vi "TTA_MATLAB_RFICSetDGAttTest.vi"(0 "Complete Settings Cluster":T2, 1 "Instrument Cluster In":T1, 5 "Sub-Function Name":string, 7 "Test Group":string, 11 "error in":errorcluster) -> (6 "SubTestSuccess":dbl[](array[numeric]), 12 "Instrument Cluster Out":T1, 15 "error out":errorcluster)   [LabVIEW 2016]
uses:
  TTA_Controls/TTA_Control_Complete_Settings_Cluster.ctl
  TTA_Controls/TTA_Control_Instrument_Cluster.ctl
  TTA_Globals/TTA_Global_Complete_Settings.vi
panel:
  out "Tx Result":cluster{"TX1":dbl[], "TXx3":dbl[]}[](array[cluster])
  out "Test Status":string
  out "DigAtt Min":dbl
  out "DigAtt Max":dbl
  out "Total RF Tx Loss (dB)":dbl
  out "Tx_Output_Power_Signal_Freq":dbl
  out "TxIF_Freq":dbl
  out "TxIF_Amp":dbl
  out "Tx IF\nOffset Array":dbl[](array[numeric])
  out "Sig Gen \nPower (dBm)":dbl
  out "Freq2":dbl
  out "BDSFreq":dbl
  out "Ref Level (dBm)":dbl
  out "RBW (Hz)":dbl
  out "Span (kHz)":dbl
  out "RFICs":i32[](array[numeric])
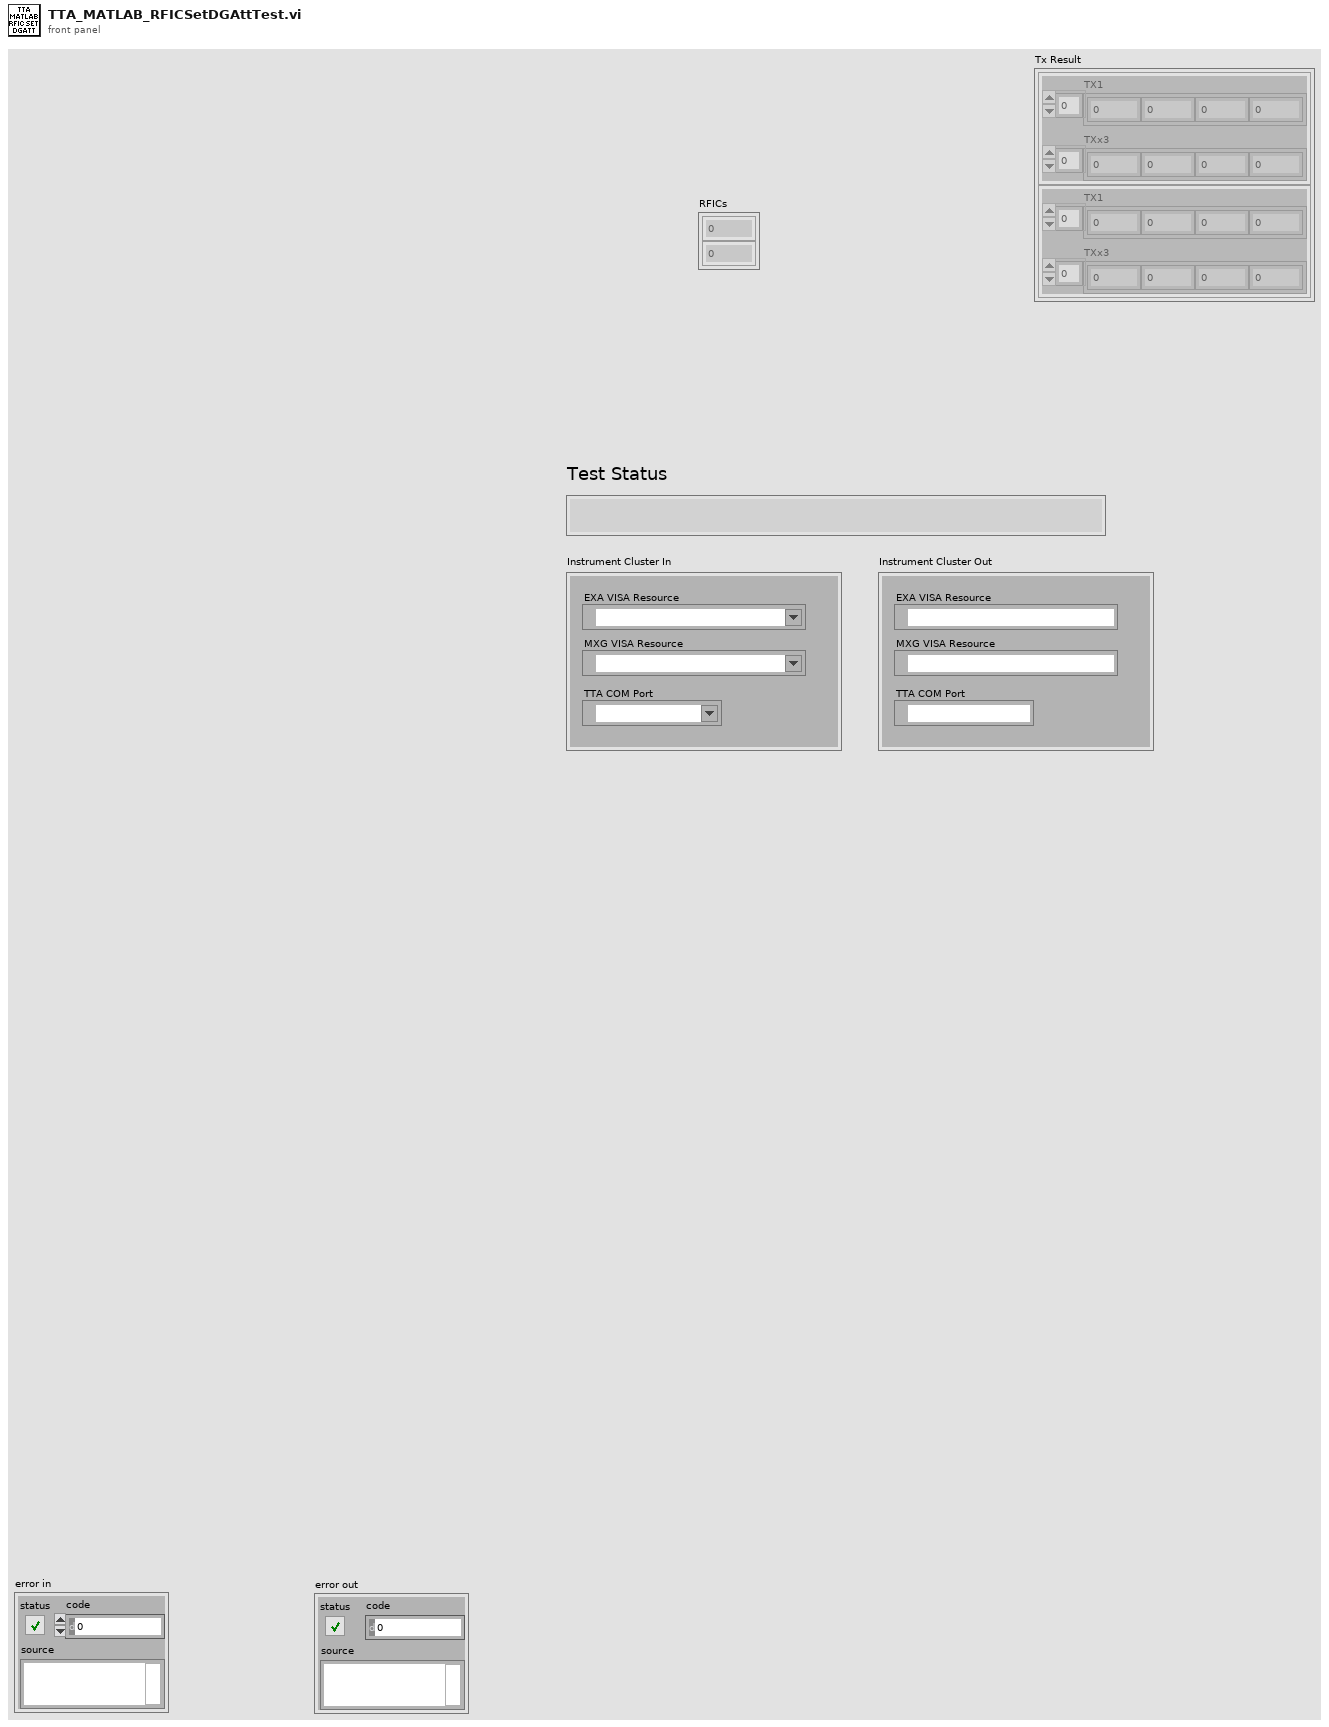
[diagram p1: front panel]
types:
  T1 = typedef "TTA_Control_Instrument_Cluster.ctl" = cluster{"EXA VISA Resource":refnum<visa-resource-name>, "MXG VISA Resource":refnum<visa-resource-name>, "TTA COM Port":refnum<visa-resource-name>}
  T2 = typedef "TTA_Control_Complete_Settings_Cluster.ctl" = cluster{"Brief Cluster":cluster{"STM Firmware File":string, "STM Firmware Address":string, "Required SW Version":string, "Template Used":string}, "Instrument Setting Cluster":cluster{"BDSFreq":dbl, "BDS Amp":dbl, "TxRFCal_Freq":dbl, "TxRFCal_Amp":dbl, "RxRFCal_Freq":dbl, "RxRFCal_Freq":dbl, "TxIF_Freq":dbl, "TxIF_Amp":dbl, "Tx_Output_Power_Signal_Freq":dbl, "Tx_ACPR_Signal_Freq":dbl, "Rx_RF_Freq":dbl, "Rx_RF_Amp":dbl, "Rx_Output_Power_Signal_Freq":dbl, "Rx_Output_Power_Sense_Freq":dbl}, "PAL Calibration\nInputs Cluster":cluster{"Amplitude Range\nMax(dBm)":dbl, "Amplitude Range\nMin(dBm)":dbl, "Amplitude Least\nCriteria (dBm)":dbl, "Frequency 1":dbl, "Frequency 2":dbl, "Frequency 3":dbl, "CAL Amplitude\nDecrement (dB)":dbl, "CAL Amplitude\nIncrement(dB)":dbl, "DownloadFile":string}, "TxOffset Cal Cluster":cluster{"Tx1 Offset (dB)":dbl, "Tx2 Offset (dB)":dbl, "Tx3 Offset (dB)":dbl, "Tx4 Offset (dB)":dbl, "Total RF Tx Loss (dB)":dbl}, "RxOffset Cal Cluster":cluster{"Rx1 Offset (dB)":dbl, "Rx2 Offset (dB)":dbl, "Rx3 Offset (dB)":dbl, "Rx4 Offset (dB)":dbl, "Total RF Rx Loss (dB)":dbl}, "TX Output Power Settings Cluster":cluster{"Frequency Sweep (MHz)":dbl[], "Sig Gen \nPower (dBm)":dbl, "Span (kHz)":dbl, "RBW (Hz)":dbl, "Ref Level (dBm)":dbl, "Low Power \nLimit":dbl, "High Power \nLimit":dbl, "DigAtt Max":dbl, "DigAtt Min":dbl}, "Tx ACPR Settings Cluster":cluster{"ACPR Filename":string, "Sampling Rate":dbl, "Power (dBm)":dbl, "IF Frequency Sweep (MHz)":dbl[], "State Name":string, "Mechanical\nAttenuation":dbl, "RefLevel Offset":dbl, "Amplitude Range\nMax (dBm)":dbl, "Amplitude Range\nMin (dBm)":dbl, "Cal Amp \nIncrement (dB)":dbl, "Cal Amp\nDecrement (dB)":dbl}, "Power Cal Cluster":cluster{"Power List (dBm)":dbl[], "Frequency (MHz)":dbl[], "Cal Decrement (dB)":dbl, "Cal Increment (dB)":dbl}, "Rx Received Power Settings Cluster":cluster{"Frequency Sweep (MHz)":dbl[], "Power (dBm)":dbl, "Span (kHz)":dbl, "RBW (Hz)":dbl, "Ref Level":dbl, "Low Power \nLimit (dBm)":dbl, "High Power\nLimit (dBm)":dbl}, "Tx Output Power Criteria Cluster":cluster{"CH1-TX1 \nMin":dbl, "CH1-TX1\nMax":dbl, "CH1-TXx3\nMin ":dbl, "CH1-TXx3\nMax":dbl, "CH2-TX1\nMin":dbl, "CH2-TX1\nMax":dbl, "CH2-TXx3\nMin":dbl, "CH2-TXx3\nMax":dbl}, "Tx ACPR Criteria Cluster":cluster{"Min Inband":dbl, "Max Close Outband":dbl, "Max Far Outband":dbl}, "Rx Output Power Criteria Cluster":cluster{"CH1-RX1 \nMin":dbl, "CH1-RX1 \nMax":dbl, "CH1-RXx3 \nMin":dbl, "CH1-RXx3\nMax":dbl, "CH2-RX1\nMin":dbl, "CH2-RX1\nMax":dbl, "CH2-RXx3\nMin":dbl, "CH2-RXx3\nMax":dbl}}
  T3 = cluster{"BDSFreq":dbl, "BDS Amp":dbl, "TxRFCal_Freq":dbl, "TxRFCal_Amp":dbl, "RxRFCal_Freq":dbl, "RxRFCal_Freq":dbl, "TxIF_Freq":dbl, "TxIF_Amp":dbl, "Tx_Output_Power_Signal_Freq":dbl, "Tx_ACPR_Signal_Freq":dbl, "Rx_RF_Freq":dbl, "Rx_RF_Amp":dbl, "Rx_Output_Power_Signal_Freq":dbl, "Rx_Output_Power_Sense_Freq":dbl}
  T4 = cluster{"Amplitude Range\nMax(dBm)":dbl, "Amplitude Range\nMin(dBm)":dbl, "Amplitude Least\nCriteria (dBm)":dbl, "Frequency 1":dbl, "Frequency 2":dbl, "Frequency 3":dbl, "CAL Amplitude\nDecrement (dB)":dbl, "CAL Amplitude\nIncrement(dB)":dbl, "DownloadFile":string}
  T5 = cluster{"Tx1 Offset (dB)":dbl, "Tx2 Offset (dB)":dbl, "Tx3 Offset (dB)":dbl, "Tx4 Offset (dB)":dbl, "Total RF Tx Loss (dB)":dbl}
  T6 = cluster{"Frequency Sweep (MHz)":dbl[], "Sig Gen \nPower (dBm)":dbl, "Span (kHz)":dbl, "RBW (Hz)":dbl, "Ref Level (dBm)":dbl, "Low Power \nLimit":dbl, "High Power \nLimit":dbl, "DigAtt Max":dbl, "DigAtt Min":dbl}
  T7 = cluster{dbl[], "TxIF_Amp":dbl, "Tx_Output_Power_Signal_Freq":dbl, "BDSFreq":dbl, "Total RF Tx Loss (dB)":dbl, "DigAtt Min":dbl, "DigAtt Max":dbl}
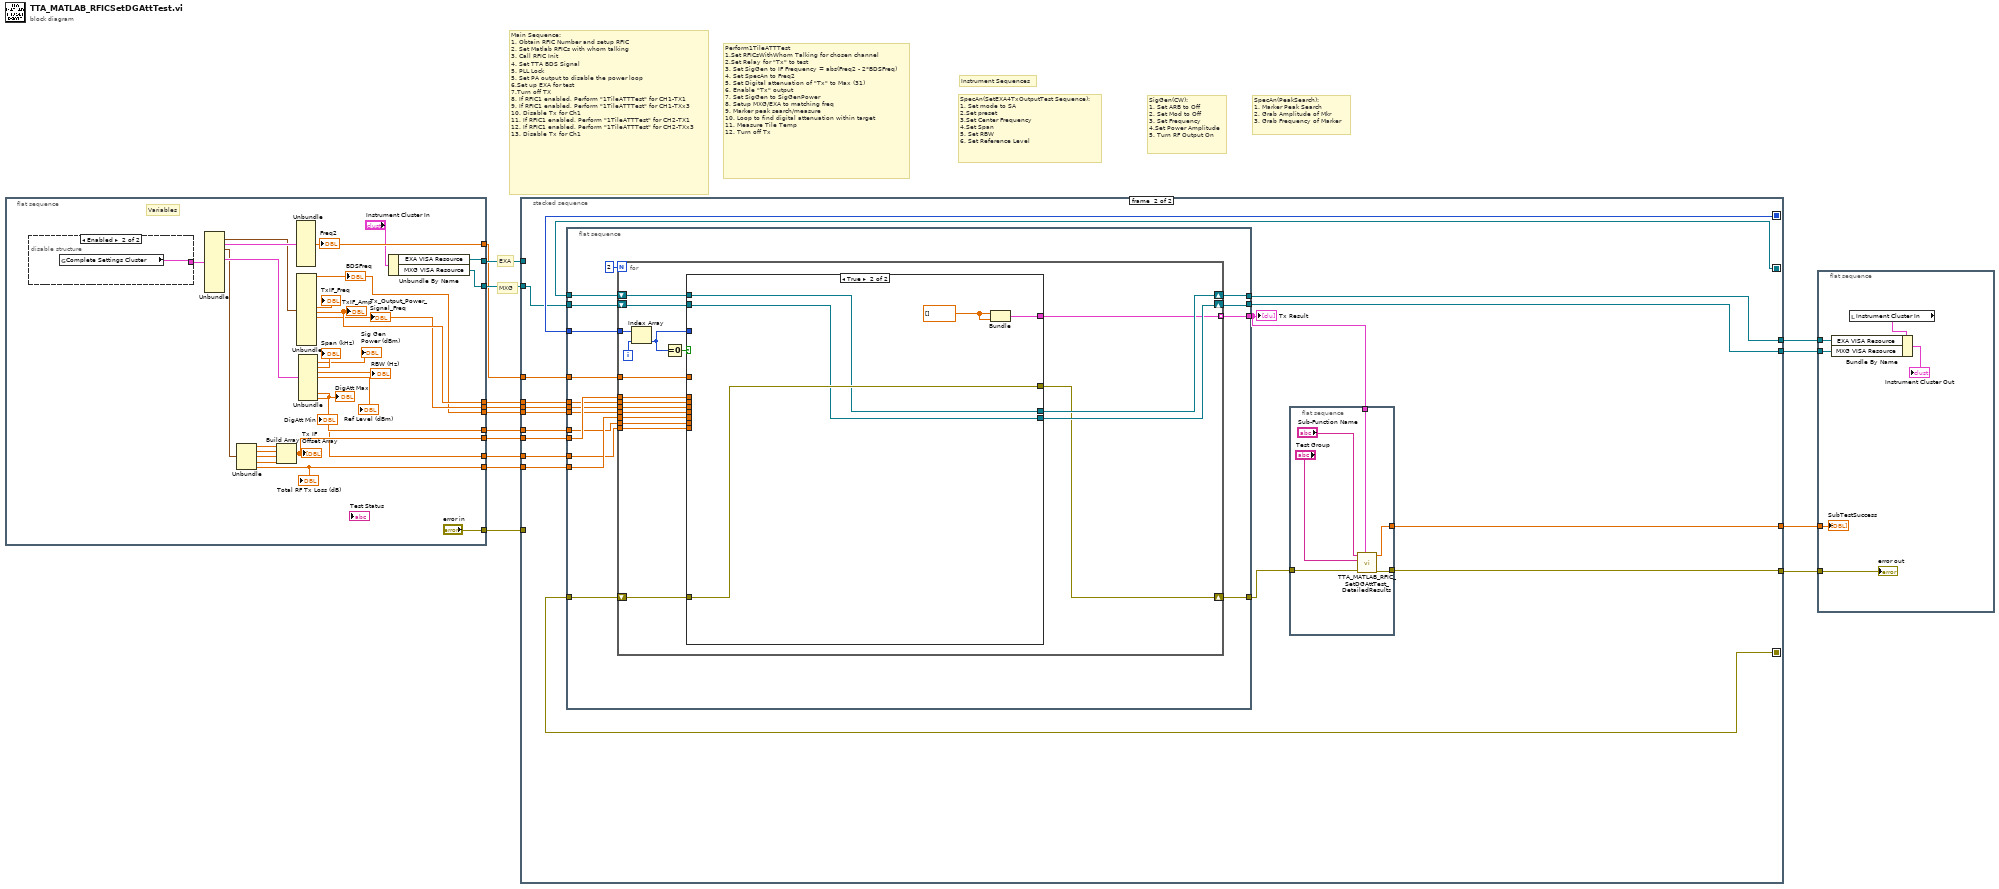
[diagram p0: block diagram]
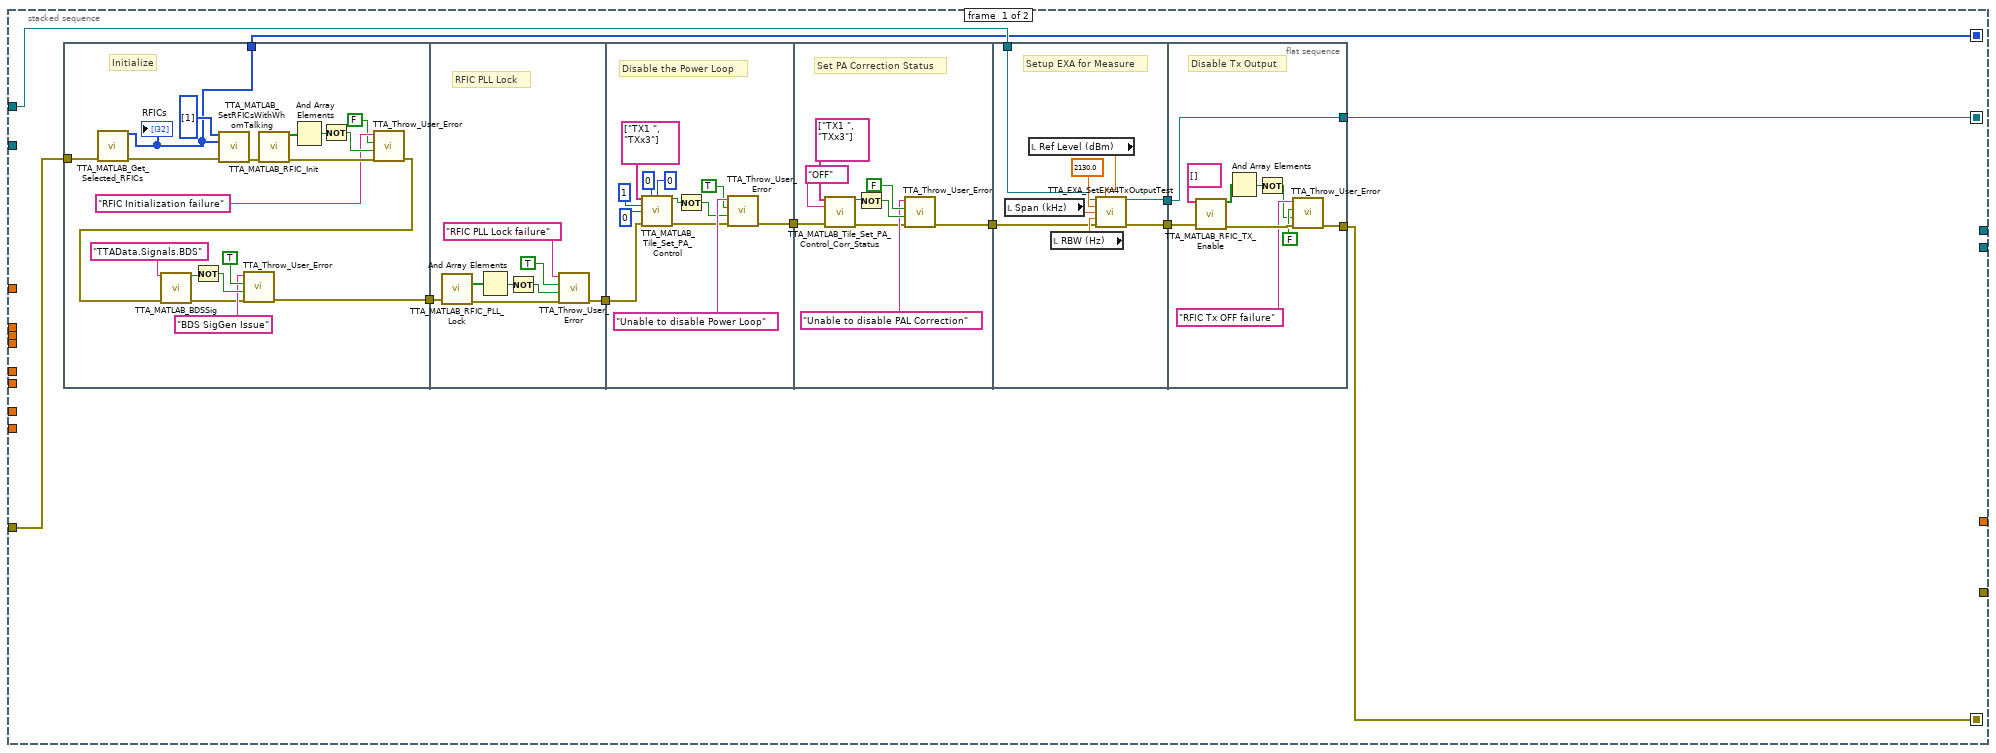
[diagram p2: hidden frame]
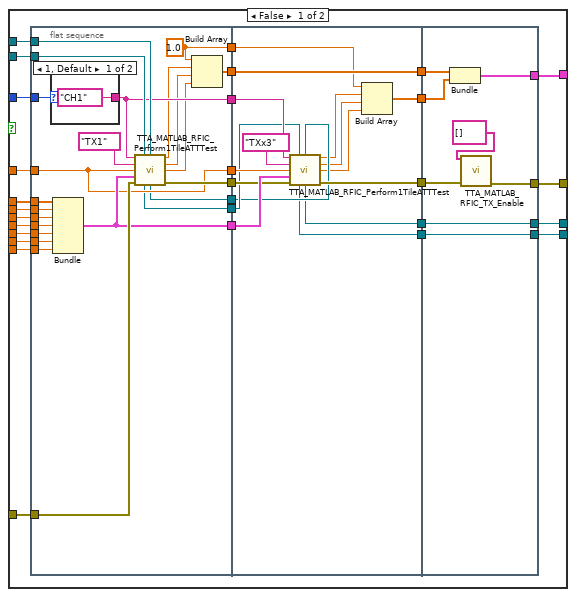
[diagram p3: hidden frame]
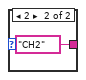
[diagram p4: hidden frame]
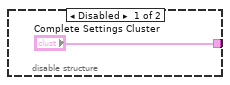
[diagram p5: hidden frame]
diagram:
  # "MXG"
  # "EXA"
  # "SpecAn(PeakSearch):\n1. Marker Peak Search\n2. Grab Amplitude of Mkr\n3. Grab Frequency of Marker"
  # "SigGen(CW):\n1. Set ARB to Off\n2. Set Mod to Off\n3. Set Frequency\n4.Set Power Amplitude\n5. Turn RF Output On"
  # "Instrument Sequences"
  # "Perform1TileATTTest\n1.Set RFICsWithWhom Talking for chosen channel\n2.Set Relay for \"Tx\" to test\n3. Set SigGen to IF Frequency = abs(Freq2 - 2*BDSFreq)\n4. Set SpecAn to Freq2\n5. Set Digital attenuation of \"Tx\" to Max (31)\n6. Enable \"Tx\" output\n7. Set SigGen to SigGenPower\n8. Setup MXG/EXA to matching freq\n9. Marker peak search/measure\n10. Loop to find digital attenuation within target\n11. Measure Tile Temp\n12. Turn off Tx"
  # "SpecAn(SetEXA4TxOutputTest Sequence):\n1. Set mode to SA\n2.Set preset\n3.Set Center Frequency\n4.Set Span\n5. Set RBW\n6. Set Reference Level"
  # "Main Sequence:\n1. Obtain RFIC Number and setup RFIC\n2. Set Matlab RFICs with whom talking\n3. Call RFIC Init\n4. Set TTA BDS Signal\n5. PLL Lock\n5. Set PA output to disable the power loop\n6.Set up EXA for test\n7.Turn off TX\n8. If RFIC1 enabled, Perform \"1TileATTTest\" for CH1-TX1\n9. If RFIC1 enabled, Perform \"1TileATTTest\" for CH1-TXx3\n10. Disable Tx for Ch1\n11. If RFIC1 enabled, Perform \"1TileATTTest\" for CH2-TX1\n12. If RFIC1 enabled, Perform \"1TileATTTest\" for CH2-TXx3\n13. Disable Tx for Ch1"
  n1 = flat-sequence {
    tunnel: ["error in"] -> w15
    tunnel: [w16] -> w14
    tunnel: [w17] -> w13
    tunnel: [w26] -> w12
    tunnel: [w25] -> w11
    tunnel: [w24] -> w10
    tunnel: [w23] -> w9
    tunnel: [w22] -> w8
    tunnel: [w21] -> w7
    tunnel: [w20] -> w6
    tunnel: [w19] -> w5
    frame #0 {
      # "Variables"
      n2 = disable-structure shown="Enabled" {
        disable-tunnel: ["Complete Settings Cluster" w43] -> w37
        frame Disabled {
        }
        frame Enabled {
          n3 = global read "TTA_Global_Complete_Settings.vi" "Complete Settings Cluster"() -> (w43:T2)
        }
      }
      n4 = Unbundle(w37) -> ("Instrument Setting Cluster"=w35:T3, "PAL Calibration\nInputs Cluster"=w36:T4, "TxOffset Cal Cluster"=w33:T5, "TX Output Power Settings Cluster"=w34:T6)  [unwired: 8 out]
      n5 = Unbundle(w33) -> ("Tx1 Offset (dB)"=w32:dbl, "Tx2 Offset (dB)"=w31:dbl, "Tx3 Offset (dB)"=w30:dbl, "Tx4 Offset (dB)"=w29:dbl, "Total RF Tx Loss (dB)"=w22:dbl)
      "Total RF Tx Loss (dB)" <- w22
      n6 = Build Array(w32, w31, w30, w29) -> (w26:dbl[])
      "Tx IF\nOffset Array" <- w26
      n7 = Unbundle(w36) -> ("Frequency 2"=w19:dbl)  [unwired: 8 out]
      "Freq2" <- w19
      n8 = Unbundle(w35) -> ("BDSFreq"=w23:dbl, "TxIF_Freq"=→"TxIF_Freq":dbl, "TxIF_Amp"=w25:dbl, "Tx_Output_Power_Signal_Freq"=w24:dbl)  [unwired: 10 out]
      "BDSFreq" <- w23
      "TxIF_Amp" <- w25
      "Tx_Output_Power_Signal_Freq" <- w24
      n9 = Unbundle(w34) -> ("Sig Gen \nPower (dBm)"=→"Sig Gen \nPower (dBm)":dbl, "Span (kHz)"=→"Span (kHz)":dbl, "RBW (Hz)"=→"RBW (Hz)":dbl, "Ref Level (dBm)"=→"Ref Level (dBm)":dbl, "DigAtt Max"=w20:dbl, "DigAtt Min"=w21:dbl)  [unwired: 3 out]
      "DigAtt Max" <- w20
      "DigAtt Min" <- w21
      n10 = Unbundle By Name("Instrument Cluster In") -> ("EXA VISA Resource"=w16:refnum<visa-resource-name>, "MXG VISA Resource"=w17:refnum<visa-resource-name>)
    }
  }
  n11 = stacked-sequence {
    seq-local: [w46 _] -> [_ w138]
    seq-local: [w45 _] -> [_ w128]
    seq-local: [w44 _] -> [_ w137]
    tunnel: w15 -> [w54 _]
    tunnel: w14 -> [w49 _]
    tunnel: w13 -> [_ w136]
    tunnel: w12 -> [_ w135]
    tunnel: w11 -> [_ w134]
    tunnel: w10 -> [_ w133]
    tunnel: w9 -> [_ w132]
    tunnel: w8 -> [_ w131]
    tunnel: w7 -> [_ w130]
    tunnel: w6 -> [_ w129]
    tunnel: w5 -> [_ w127]
    tunnel: [_ w123] -> w4
    tunnel: [_ w126] -> w3
    tunnel: [_ w125] -> w2
    tunnel: [_ w122] -> w1
    frame #0 {
      n12 = flat-sequence {
        tunnel: w54 -> [w71]
        tunnel: [w56] -> w53
        tunnel: [w55] -> w46
        tunnel: w53 -> [w81]
        tunnel: [w76] -> w52
        tunnel: w52 -> [w88]
        tunnel: [w82] -> w51
        tunnel: w51 -> [w100]
        tunnel: [w94] -> w50
        tunnel: w50 -> [w106]
        tunnel: w49 -> [w105]
        tunnel: [w104] -> w48
        tunnel: [w103] -> w47
        tunnel: [w120] -> w44
        tunnel: w48 -> [w120]
        tunnel: w47 -> [w118]
        tunnel: [w111] -> w45
        frame #0 {
          # "Initialize"
          n13 = call "TTA_MATLAB_Get_Selected_RFICs.vi"("error in"=w71) -> ("RFICs"=w55:i32[], "error out"=w72:errorcluster)  [unwired: 13 in]
          "RFICs" <- w55
          n14 = call "TTA_MATLAB_SetRFICsWithWhomTalking.vi"("Panel Array"=i32[] [1], "RFIC Array"=w55, "error in"=w72) -> ("error out"=w70:errorcluster)  [unwired: 12 in]
          n15 = call "TTA_MATLAB_RFIC_Init.vi"("error in"=w70) -> ("SuccessComm"=w68:bool[], "error out"=w69:errorcluster)  [unwired: 13 in]
          n16 = And Array Elements(Boolean array=w68) -> (logical AND=w67:bool)
          n17 = Not(x=w67) -> (.not. x?=w66:bool)
          n18 = call "TTA_Throw_User_Error.vi"("error in"=w69, "Error?"=w66, "Stop Execution on Fail"=FALSE, "Error Message"="RFIC Initialization failure") -> ("error out"=w62:errorcluster)  [unwired: 7 in]
          n19 = call "TTA_MATLAB_BDSSig.vi"("Signal Settings"="TTAData.Signals.BDS", "error in"=w62) -> ("Success"=w61:bool, "error out"=w57:errorcluster)  [unwired: 12 in]
          n20 = Not(x=w61) -> (.not. x?=w60:bool)
          n21 = call "TTA_Throw_User_Error.vi"("error in"=w57, "Error?"=w60, "Stop Execution on Fail"=TRUE, "Error Message"="BDS SigGen Issue") -> ("error out"=w56:errorcluster)  [unwired: 7 in]
        }
        frame #1 {
          # "RFIC PLL Lock"
          n22 = call "TTA_MATLAB_RFIC_PLL_Lock.vi"("error in"=w81) -> ("SuccessComm"=w80:bool[], "error out"=w77:errorcluster)  [unwired: 11 in, 2 out]
          n23 = And Array Elements(Boolean array=w80) -> (logical AND=w75:bool)
          n24 = Not(x=w75) -> (.not. x?=w74:bool)
          n25 = call "TTA_Throw_User_Error.vi"("error in"=w77, "Error?"=w74, "Stop Execution on Fail"=TRUE, "Error Message"="RFIC PLL Lock failure") -> ("error out"=w76:errorcluster)  [unwired: 7 in]
        }
        frame #2 {
          # "Disable the Power Loop"
          n26 = call "TTA_MATLAB_Tile_Set_PA_Control.vi"("Channels"=string[] ["TX1 ", "TXx3"], "OutPower"=0, "InPower"=0, "Temp"=1, "Current"=0, "error in"=w88) -> ("Success"=w85:bool, "error out"=w83:errorcluster)  [unwired: 6 in, 2 out]
          n27 = Not(x=w85) -> (.not. x?=w84:bool)
          n28 = call "TTA_Throw_User_Error.vi"("error in"=w83, "Error?"=w84, "Stop Execution on Fail"=TRUE, "Error Message"="Unable to disable Power Loop") -> ("error out"=w82:errorcluster)  [unwired: 7 in]
        }
        frame #3 {
          # "Set PA Correction Status"
          n29 = call "TTA_MATLAB_Tile_Set_PA_Control_Corr_Status.vi"("Channels"=string[] ["TX1 ", "TXx3"], "ModeAdapt"="OFF", "error in"=w100) -> ("Success"=w98:bool, "error out"=w95:errorcluster)  [unwired: 9 in, 2 out]
          n30 = Not(x=w98) -> (.not. x?=w97:bool)
          n31 = call "TTA_Throw_User_Error.vi"("error in"=w95, "Error?"=w97, "Stop Execution on Fail"=FALSE, "Error Message"="Unable to disable PAL Correction") -> ("error out"=w94:errorcluster)  [unwired: 7 in]
        }
        frame #4 {
          # "Setup EXA for Measure"
          n32 = local read "Span (kHz)"() -> (w109:dbl)
          n33 = local read "Ref Level (dBm)"() -> (w108:dbl)
          n34 = local read "RBW (Hz)"() -> (w107:dbl)
          n35 = call "TTA_EXA_SetEXA4TxOutputTest.vi"("VISA resource In"=w105, "Reference Level (dBm)"=w108, "Frequency (MHz)"=2130.0, "Span (kHz)"=w109, "RBW (Hz)"=w107, "error in"=w106) -> ("VISA resource Out"=w104:refnum<visa-resource-name>, "error out"=w103:errorcluster)  [unwired: 8 in]
        }
        frame #5 {
          # "Disable Tx Output"
          n36 = call "TTA_MATLAB_RFIC_TX_Enable.vi"("Channels"=string[] [], "error in"=w118) -> ("SuccessComm"=w113:bool[], "error out"=w117:errorcluster)  [unwired: 12 in]
          n37 = And Array Elements(Boolean array=w113) -> (logical AND=w114:bool)
          n38 = Not(x=w114) -> (.not. x?=w112:bool)
          n39 = call "TTA_Throw_User_Error.vi"("error in"=w117, "Error?"=w112, "Stop Execution on Fail"=FALSE, "Error Message"="RFIC Tx OFF failure") -> ("error out"=w111:errorcluster)  [unwired: 7 in]
        }
      }
    }
    frame #1 {
      n40 = flat-sequence {
        tunnel: w138 -> [w161]
        tunnel: w137 -> [w160]
        tunnel: w136 -> [w159]
        tunnel: w135 -> [w158]
        tunnel: w134 -> [w157]
        tunnel: w133 -> [w156]
        tunnel: w132 -> [w155]
        tunnel: w131 -> [w154]
        tunnel: w130 -> [w153]
        tunnel: w129 -> [w152]
        tunnel: w128 -> [w151]
        tunnel: w127 -> [w150]
        tunnel: [w149] -> w125
        tunnel: [w148] -> w126
        tunnel: [w147] -> w124
        tunnel: [w145] -> w121
        frame #0 {
          n41 = for {
            N: 2 -> [_]
            tunnel: w161 -> [w166]
            tunnel: w158 -> [w178]
            tunnel: w157 -> [w177]
            tunnel: w156 -> [w176]
            tunnel: w155 -> [w175]
            tunnel: w154 -> [w174]
            tunnel: w153 -> [w173]
            tunnel: w152 -> [w172]
            tunnel: w150 -> [w170]
            shift-right: [w169] -> w148
            shift-left: w160 -> [w180]
            shift-right: [w168] -> w149
            shift-left: w159 -> [w179]
            shift-right: [w167] -> w147
            shift-left: w151 -> [w171]
            tunnel: [w162] -> w145 mode=indexing
            i -> [w165]
            n42 = Index Array(array=w166, index=w165) -> (element=w164:i32)
            n43 = Equal To 0?(x=w164) -> (x = 0?=w163:bool)
            n44 = case shown="True" w163 {
              tunnel: w180 -> [w200 w260]
              tunnel: w179 -> [w199 w259]
              tunnel: w178 -> [w198 _]
              tunnel: w177 -> [w197 _]
              tunnel: w176 -> [w196 _]
              tunnel: w175 -> [w195 _]
              tunnel: w174 -> [w194 _]
              tunnel: w173 -> [w193 _]
              tunnel: w172 -> [w192 _]
              tunnel: w171 -> [w191 w263]
              tunnel: w170 -> [w190 _]
              tunnel: [w181 w262] -> w162
              tunnel: [w189 w260] -> w169
              tunnel: [w188 w259] -> w168
              tunnel: [w187 w263] -> w167
              tunnel: w164 -> [w186 _]
              frame False {
                n45 = flat-sequence {
                  tunnel: w186 -> [w215]
                  tunnel: w200 -> [w231]
                  tunnel: w199 -> [w230]
                  tunnel: w198 -> [w229]
                  tunnel: w197 -> [w228]
                  tunnel: w196 -> [w227]
                  tunnel: w195 -> [w226]
                  tunnel: w194 -> [w225]
                  tunnel: w193 -> [w224]
                  tunnel: w192 -> [w223]
                  tunnel: w191 -> [w222]
                  tunnel: [w221] -> w209
                  tunnel: [w220] -> w208
                  tunnel: [w219] -> w207
                  tunnel: w190 -> [w218]
                  tunnel: [w218] -> w206
                  tunnel: [w217] -> w205
                  tunnel: [w216] -> w204
                  tunnel: [w211] -> w185
                  tunnel: [w210] -> w183
                  tunnel: w209 -> [w249]
                  tunnel: w208 -> [w248]
                  tunnel: w207 -> [w247]
                  tunnel: w206 -> [w246]
                  tunnel: w205 -> [w244]
                  tunnel: w204 -> [w243]
                  tunnel: [w245] -> w203
                  tunnel: [w242] -> w202
                  tunnel: [w241] -> w201
                  tunnel: w185 -> [w240]
                  tunnel: [w240] -> w184
                  tunnel: w183 -> [w239]
                  tunnel: [w235] -> w182
                  tunnel: [w257] -> w189
                  tunnel: [w258] -> w188
                  tunnel: w203 -> [w255]
                  tunnel: w202 -> [w258]
                  tunnel: w201 -> [w257]
                  tunnel: [w254] -> w187
                  tunnel: w184 -> [w253]
                  tunnel: w182 -> [w252]
                  tunnel: [w251] -> w181
                  frame #0 {
                    w210 = 1.0
                    n46 = case shown="1, Default" w215 {
                      tunnel: ["CH1" ("Channel") "CH2" ("Channel")] -> w221
                      frame 1, Default {
                      }
                      frame 2 {
                      }
                    }
                    n47 = Bundle(w229, "TxIF_Amp"=w228, "Tx_Output_Power_Signal_Freq"=w227, "BDSFreq"=w226, "Total RF Tx Loss (dB)"=w225, "DigAtt Min"=w224, "DigAtt Max"=w223) -> (w220:T7)  [unwired: 1 in]
                    n48 = call "TTA_MATLAB_RFIC_Perform1TileATTTest.vi"("Channel"=w221, "MXG VISA Resource In"=w230, "EXA VISA Resource"=w231, "Tx"="TX1", "Freq_Cal_List"=w218, "DigATT Values"=w220, "error in"=w222) -> ("Amp"=w214:dbl, "Attenuation"=w213:dbl, "Temp"=w212:dbl, "MXG VISA Resource Out"=w217:refnum<visa-resource-name>, "EXA VISA Resource Out"=w216:refnum<visa-resource-name>, "error out"=w219:errorcluster)  [unwired: 3 in]
                    n49 = Build Array(w210, w214, w213, w212) -> (w211:dbl[])
                  }
                  frame #1 {
                    n50 = call "TTA_MATLAB_RFIC_Perform1TileATTTest.vi"("Channel"=w249, "MXG VISA Resource In"=w244, "EXA VISA Resource"=w243, "Tx"="TXx3", "Freq_Cal_List"=w246, "DigATT Values"=w248, "error in"=w247) -> ("Amp"=w238:dbl, "Attenuation"=w237:dbl, "Temp"=w236:dbl, "MXG VISA Resource Out"=w242:refnum<visa-resource-name>, "EXA VISA Resource Out"=w241:refnum<visa-resource-name>, "error out"=w245:errorcluster)  [unwired: 3 in]
                    n51 = Build Array(w239, w238, w237, w236) -> (w235:dbl[])
                  }
                  frame #2 {
                    n52 = Bundle(w253, w252) -> (w251:cluster{dbl[], dbl[]})  [unwired: 1 in]
                    n53 = call "TTA_MATLAB_RFIC_TX_Enable.vi"("Channels"=string[] [], "error in"=w255) -> ("error out"=w254:errorcluster)  [unwired: 12 in, 1 out]
                  }
                }
              }
              frame True {
                w261 = dbl[] []
                n54 = Bundle(w261, w261) -> (w262:cluster{dbl[], dbl[]})  [unwired: 1 in]
              }
            }
          }
        }
      }
      n55 = flat-sequence {
        tunnel: w124 -> [w139]
        tunnel: [w144] -> w123
        tunnel: [w143] -> w122
        tunnel: w121 -> [w142]
        frame #0 {
          n56 = call "TTA_MATLAB_RFIC_SetDGAttTest_DetailedResults.vi"("Tx Result"=w142, "error in"=w139, "TestGroup"="Test Group", "SubTest"="Sub-Function Name") -> ("error out"=w144:errorcluster, "SubTestSuccess"=w143:dbl[])  [unwired: 6 in]
        }
      }
      "Tx Result" <- w121
    }
  }
  n57 = flat-sequence {
    tunnel: w4 -> [w269]
    tunnel: w3 -> [w266]
    tunnel: w2 -> [w265]
    tunnel: w1 -> [w264]
    frame #0 {
      n58 = local read "Instrument Cluster In"() -> (w267:T1)
      n59 = Bundle By Name(cluster=w267, "EXA VISA Resource"=w266, "MXG VISA Resource"=w265) -> (→"Instrument Cluster Out":T1)
      "error out" <- w269
      "SubTestSuccess" <- w264
    }
  }
